vi "XY_GetCenterOfMass.vi"(10 "Image in":u8[][](array[numeric])) -> (0 "center-based coordinates (pix)":dbl[](array[numeric]), 1 "median image":dbl format="%0.2f", 2 "corner-based Coordinates (pix)":dbl[](array[numeric]) format="%.2f")   [LabVIEW 2011]
uses:
  <vilib>/Analysis/NI_AALBase.lvlib
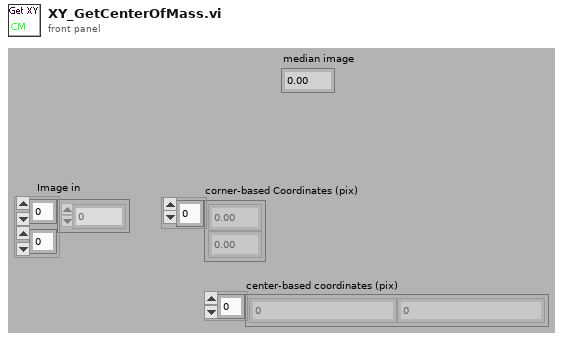
[diagram p1: front panel]
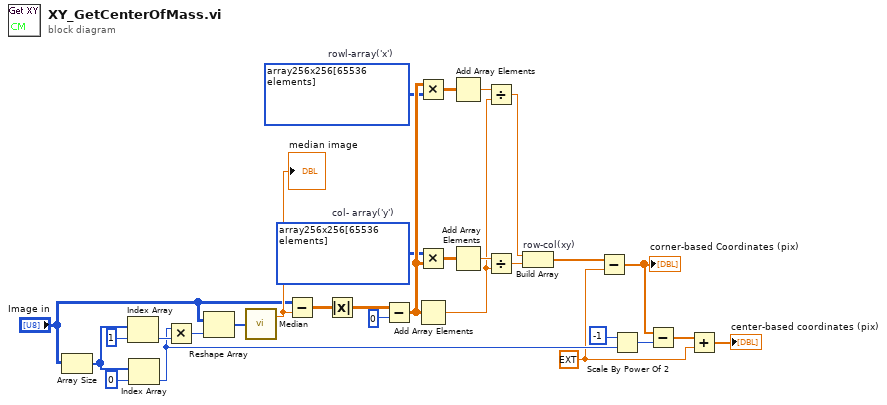
[diagram p0: block diagram]
diagram:
  w2 = ext 0.0 ("y")
  w1 = i32[][] array256x256[65536 elements]  # rowl-array('x')
  w19 = i32[][] array256x256[65536 elements]  # col- array('y')
  n1 = Array Size(array="Image in") -> (size(s)=w9:i32[])
  n2 = Index Array(array=w9, index=1 ("Index")) -> (element=w17:i32)
  n3 = Index Array(array=w9, index=0) -> (element=w7:i32)
  n4 = Multiply(x=w7, y=w17) -> (x*y=w16:i32)
  n5 = Reshape Array("Image in", w16) -> (w15:u8[])
  n6 = call <vilib>:"Median.vi"("X"=w15) -> ("median"=w14:dbl)  [unwired: 1 out]
  "median image" <- w14
  n7 = Subtract(x="Image in", y=w14) -> (x-y=w22:dbl[][])
  n8 = Absolute Value(x=w22) -> (abs(x)=w13:dbl[][])
  n9 = Subtract(x=w13, y=0) -> (x-y=w20:dbl[][])
  n10 = Multiply(x=w20, y=w1) -> (x*y=w29:dbl[][])
  n11 = Multiply(x=w19, y=w20) -> (x*y=w28:dbl[][])
  n12 = Add Array Elements(numeric array=w20) -> (sum=w25:dbl)
  n13 = Add Array Elements(numeric array=w29) -> (sum=w26:dbl)
  n14 = Add Array Elements(numeric array=w28) -> (sum=w27:dbl)
  n15 = Divide(x=w26, y=w25) -> (x/y=w23:dbl)
  n16 = Divide(x=w27, y=w25) -> (x/y=w24:dbl)
  n17 = Build Array "row-col(xy)"(w23, w24) -> (w11:dbl[])
  n18 = Subtract(x=w11, y=w2) -> (x-y=w5:ext[])
  "corner-based Coordinates (pix)" <- w5
  n19 = Scale By Power Of 2(n=i16 -1, x=w7) -> (x*2^n=w6:i32)
  n20 = Subtract(x=w5, y=w6) -> (x-y=w4:ext[])
  n21 = Add(x=w4, y=w2) -> (x+y=→"center-based coordinates (pix)":ext[])
